vi "HelperVI1.vi"() -> ()   [LabVIEW 2016, in "test_ValueSignal.lvlib"]
uses:
  test_ValueSignal.lvlib
panel:
  in  "Cluster":T1
  in  "String":string
  out "Boolean":bool
  in  "Numeric":dbl
  in  "Tab Control":enum32{"Page 1", "Page 2", "Page 3"}(tab)
  in  "Numeric_tab":dbl
  out "Boolean_tab":bool
  in  "String_tab":string
  in  "Cluster_tab":T2
  in  "BigCluster_tab":T3
  in  "BigCluster":T3
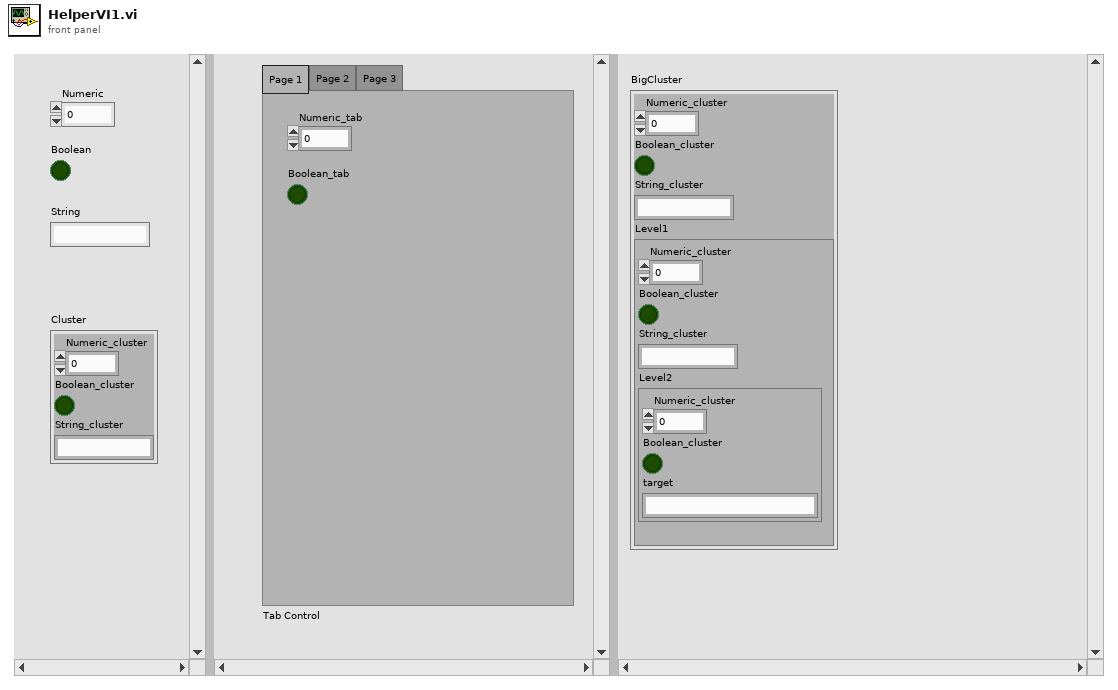
[diagram p1: front panel]
types:
  T1 = cluster{"Numeric_cluster":dbl, "Boolean_cluster":bool, "String_cluster":string}
  T2 = cluster{"Numeric_cluster_tab":dbl, "Boolean_cluster_tab":bool, "String_cluster_tab":string}
  T3 = cluster{"Numeric_cluster":dbl, "Boolean_cluster":bool, "String_cluster":string, "Level1":cluster{"Numeric_cluster":dbl, "Boolean_cluster":bool, "String_cluster":string, "Level2":cluster{"Numeric_cluster":dbl, "Boolean_cluster":bool, "target":string}}}
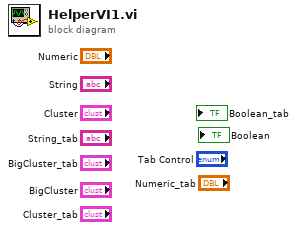
[diagram p0: block diagram]
diagram:
